vi "3_2_Face_Detection_Inference(CPU,GPU,RT)(File).vi"() -> ()   [LabVIEW 2020]
doc: "This example demonstrates the usage of the \"DeepLTK FPGA Addon\" for deploying a Face Detection model on a PXI-FPGA board, utilizing an input image sourced from a file.\n\nMore Examples: https://github.com/ngenehub/deepltk_fpga_examples"
uses:
  <vilib>/Ngene/Deep Learning Toolkit/Toolkit/NN_Network/Controls/NN_Device.ctl
  <vilib>/Ngene/Deep Learning Toolkit/Toolkit/NN_Network/Controls/NN_Save_Before_Destroy_Options.ctl
  6caafd12-b030-411a-8c32-73dfdbcc6777.vi
  <vilib>/Ngene/Deep Learning Toolkit/Toolkit/Utils/Vision/Coords_Rect2PolyLine.vi
  <vilib>/Ngene/Deep Learning Toolkit/Toolkit/NN_Network/API/NN_Set_Input/3D/NN_Set_Input(3D_SGL_idx).vi
  <vilib>/vision/NI_Vision_Development_Module.lvlib
  <vilib>/Ngene/Deep Learning Toolkit/Toolkit/Deep_Learning_Toolkit_by_Ngene.lvlib
  <vilib>/ptbypt/NI_PtbyPt.lvlib
panel:
  out "Loop time":dbl=0.10532894999996642 format="%#_4p"
  in  "NN_Device":T1
  out "Display":T2(plugin-control)
  out "Inference time":dbl=0.09766583999989961 format="%#_4p"
  out "Sample Path":path=path "D:/Ngene/GitHub/deepltk_fpga_examples/2_Face_Detection(PXI,sbRIO)/Dataset/Images/8_Election_Campain_Election_Campaign_8_529.jpg"
  in  "Select Sample":i32=19 min=0 max=19 step=1
  in  "Dataset Path (Images)":path=path "D:/Ngene/GitHub/deepltk_fpga_examples/2_Face_Detection(PXI,sbRIO)/Dataset/Images"
  in  "Confidence_Thresh":sgl=0.4
  in  "IOU_Thresh":sgl=0.3
  in  "Stop":bool
  in  "Weight File Path":path=path "D:/Ngene/GitHub/deepltk_fpga_examples/2_Face_Detection(PXI,sbRIO)/Models/Face_Detection_Original/Face_Detection.bin"
  in  "Configuration File Path":path=path "D:/Ngene/GitHub/deepltk_fpga_examples/2_Face_Detection(PXI,sbRIO)/Models/Face_Detection_Original/Face_Detection.cfg"
  # "Overview: \nOverview:  This example demonstrates usage of Deep Learning Toolkit for deploying a Face Detection model, utilizing an input image sourced from a file.\nRequirements: \n•DeepLTK - Deep Learning Toolkit for LabVIEW (https://www.ngene.co/deep-learning-toolkit-for-labview)\n• NI Vision Development Module"
  # "Instructions:\nNote: To run the example on an RT target, copy the pretrained model and test images to the RT target.\n1. Provide the \"Network Configuration File Path\" and \"Weight File Path\" locted in \"Models\\Face_Detection_Original\" folder in the project.\n2.\tProvide the path to the folder with test images in the \"Dataset Path (Images)\" control. A sample is available in the \"Dataset\" folder. \n3. Use NN_Device to specify the device (CPU or GPU) for execution. GPU is applicable only for 64-bit LabVIEW.\n4. Run the VI. \n5. Observe the detections drawn on the \"Display\". The info on the top left of each bounding box represents detected object class and the confidence level.  \n4. Change \"Select Sample\" value to select different image samples from the datset.\n5. Hit \"Stop\" button to stop the VI\nMore Examples:  https://github.com/ngenehub/deepltk_examples"
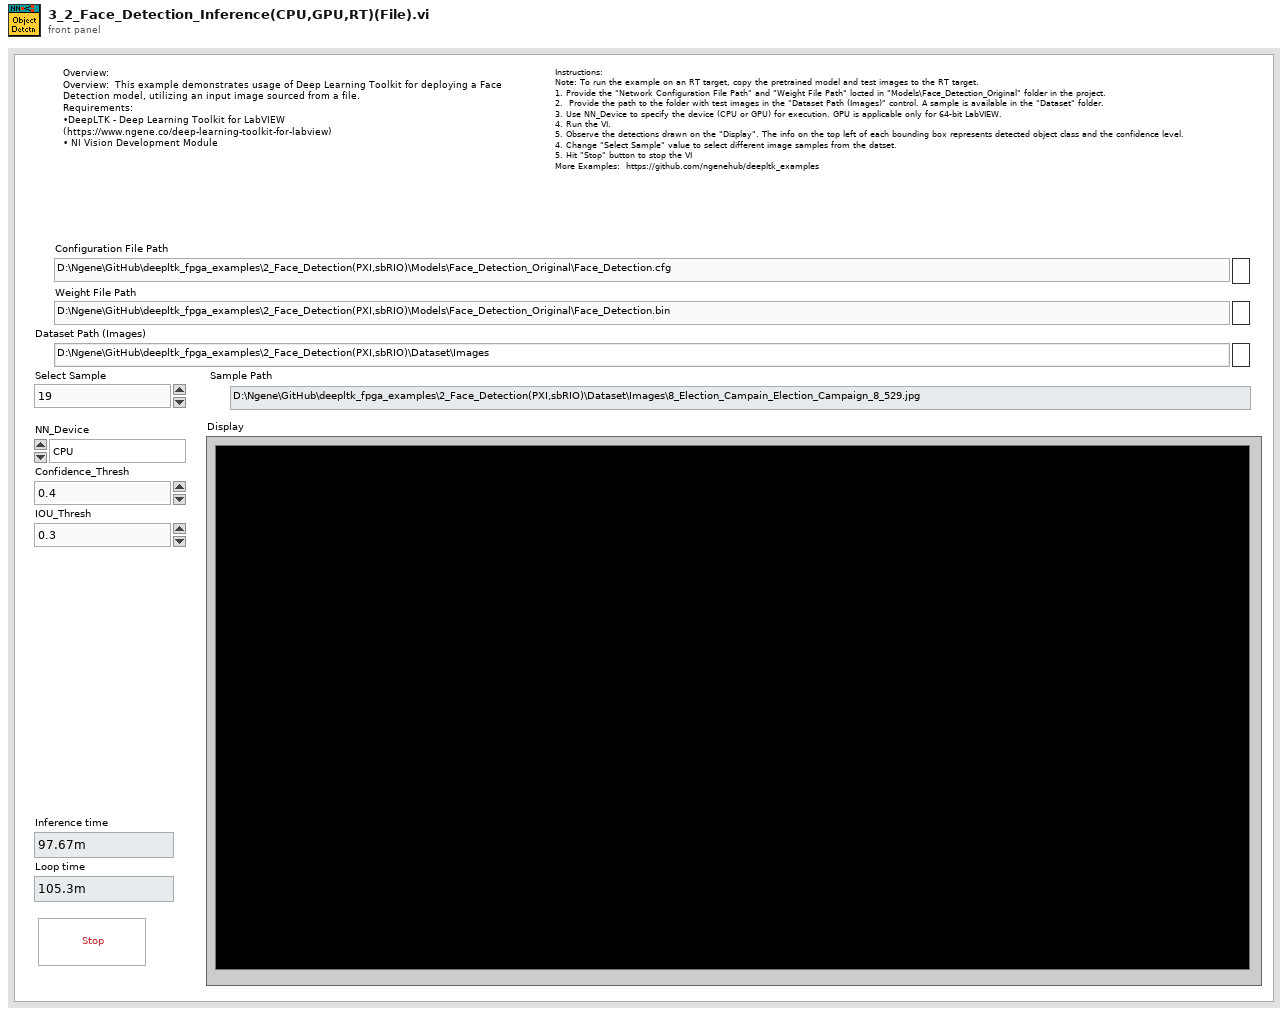
[diagram p1: front panel]
types:
  T1 = typedef "Deep_Learning_Toolkit_by_Ngene.lvlib/NN_Device.ctl" = enum16{"CPU", "GPU"}
  T2 = typedef "IMAQ Image.ctl" = refnum<image>
  T3 = typedef "Image Type" = u32
  T4 = typedef "Deep_Learning_Toolkit_by_Ngene.lvlib/NN_Save_Before_Destroy_Options.ctl" = cluster{"CFG?":bool, "Weights?":bool, "Render?":bool}
  T5 = typedef "Deep_Learning_Toolkit_by_Ngene.lvlib/NN_Config_Params.ctl" = cluster{"Name":string, "mBatch":i32, "NN_Train_Params":T6, "LR_Decay_Policy":T9, "Labels":string[], "Loss":T11}
  T6 = typedef "Deep_Learning_Toolkit_by_Ngene.lvlib/NN_Train_Params.ctl" = cluster{"Optimizer":T7, "Beta_1":sgl, "Beta_2":sgl, "Weight Decay(L1)":sgl, "Weight Decay(L2)":sgl, "Data_Sampling":T8}
  T7 = typedef "Deep_Learning_Toolkit_by_Ngene.lvlib/NN_Train_Optimizer.ctl" = enum16{"SGD", "Adam", "Adagrad", "Adadelta", "RMSProp", "Nesterov"}
  T8 = typedef "Deep_Learning_Toolkit_by_Ngene.lvlib/NN_Train_Data_Sampling.ctl" = enum16{"Random", "Sequential"}
  T9 = typedef "Deep_Learning_Toolkit_by_Ngene.lvlib/NN_LR_Policy_Cfg.ctl" = cluster{"Policy_Type":T10, "LR0":dbl, "k":sgl, "WarmUp_Policy":enum16{"Step", "Ramp"}, "WarmUp_Iter":i32, "WarmUp_Ratio":sgl}
  T10 = typedef "Deep_Learning_Toolkit_by_Ngene.lvlib/NN_LR_Policy_Type.ctl" = enum16{"Manual", "Step", "Exp", "1/t"}
  T11 = typedef "Deep_Learning_Toolkit_by_Ngene.lvlib/NN_Loss_Config_Params.ctl" = cluster{"Loss_Type":T12, "Loss_Conf_Params":variant}
  T12 = typedef "Deep_Learning_Toolkit_by_Ngene.lvlib/NN_Loss_Type.ctl" = enum16{"None", "MSE", "CrossEntropy", "YOLO_v2", "YOLO_v4"}
  T13 = typedef "Deep_Learning_Toolkit_by_Ngene.lvlib/NN_Layer_Config_Params.ctl" = cluster{"Layer_Type":T14, "Layer_Conf_Params":variant, "Input Layers":string[]}
  T14 = typedef "Deep_Learning_Toolkit_by_Ngene.lvlib/NN_Layer_Type.ctl" = enum16{"Input1D", "Input3D", "Conv1D", "Conv2D", "Conv2D_Adv", "MaxPool", "AvgPool", "UpSample", "DropOut3D", "ShortCut", "Concat", "SoftMax3D", "FC", "DropOut", "Softmax", "Flatten", "YOLO_v2", "YOLO_v4", "Activation", "BatchNormalization", "Unsupported"}
  T15 = typedef "Deep_Learning_Toolkit_by_Ngene.lvlib/NN.ctl" = cluster{"Name":string, "No of Layers":i32, "mBatch":i32, "Layers":T16[], "Dimty":T17, "Dims_In":T18, "Dims_Out":T18, "Working_Dir":path, "Train?":bool, "Train_Params":T6, "LR_Update_Policy":T9, "Session Data":T19, "Ground_truth":T20, "NNg_hdls":T21, "NN_Device":T1, "GPU Id":i32, "Labels":string[], "Receptive Field":T22[], "Loss_Type":T12, "Loss_Cfg_Prms":variant, "NNG_WS":T23}
  T16 = typedef "Deep_Learning_Toolkit_by_Ngene.lvlib/NN_Layer_ref.ctl" = refnum<data-value>
  T17 = typedef "Deep_Learning_Toolkit_by_Ngene.lvlib/NN_In_Out_Dim-ty.ctl" = enum8{"In1D_Out1D", "In3D_Out1D", "In3D_Out3D", "In3D_OutBBox"}
  T18 = typedef "Deep_Learning_Toolkit_by_Ngene.lvlib/NN_Dims(C,H,W).ctl" = cluster{"C":i32, "H":i32, "W":i32}
  T19 = typedef "Deep_Learning_Toolkit_by_Ngene.lvlib/NN_Train_Session_Data.ctl" = cluster{"Epochs":sgl, "Tot_Iter":i32, "LR":sgl, "LR_iter":i32}
  T20 = typedef "Deep_Learning_Toolkit_by_Ngene.lvlib/NN_Ground_truth.ctl" = cluster{"Y":variant}
  T21 = typedef "Deep_Learning_Toolkit_by_Ngene.lvlib/nng_cuda_handles.ctl" = cluster{"cudnn":u64, "cublas":u64, "stream":u64, "curand":u64}
  T22 = typedef "Deep_Learning_Toolkit_by_Ngene.lvlib/NN_Dims(V,H).ctl" = cluster{"V":i32, "H":i32}
  T23 = typedef "Deep_Learning_Toolkit_by_Ngene.lvlib/NNG_WS.ctl" = cluster{"NNG_WS_Mem":T24, "Max_WS_Size":i64}
  T24 = typedef "Deep_Learning_Toolkit_by_Ngene.lvlib/NNg_WS_Mem_DVR.ctl" = refnum<data-value>
  T25 = typedef "Deep_Learning_Toolkit_by_Ngene.lvlib/NN_Layer.ctl" = cluster{"Name":string, "Layer_Data":variant, "Layer_Type":T14, "Dims_In":T18, "Layers_In":variant, "Dims_Out":T18, "Layers_Out":variant, "Metrics":T26, "GPU_Data":variant, "mBatch":i32, "NN_Device":T1, "NNg_hdls":T21, "Train?":bool, "Dimty":T27, "RecptField":T28}
  T26 = typedef "Deep_Learning_Toolkit_by_Ngene.lvlib/NN_Layer_Metrics.ctl" = cluster{"Data":dbl, "Params":dbl, "Ops":dbl}
  T27 = typedef "Deep_Learning_Toolkit_by_Ngene.lvlib/NN_Layer_Dimty.ctl" = enum16{"1D", "3D"}
  T28 = typedef "Deep_Learning_Toolkit_by_Ngene.lvlib/NN_Layer_RF_State.ctl" = cluster{"Dims":T22, "J":T22}
  T29 = typedef "Deep_Learning_Toolkit_by_Ngene.lvlib/NN_BBox_Detection.ctl" = cluster{"Class":i32, "Conf Level":sgl, "BBox":T30}
  T30 = typedef "Deep_Learning_Toolkit_by_Ngene.lvlib/NN_BBox.ctl" = cluster{"x":sgl, "y":sgl, "w":sgl, "h":sgl}
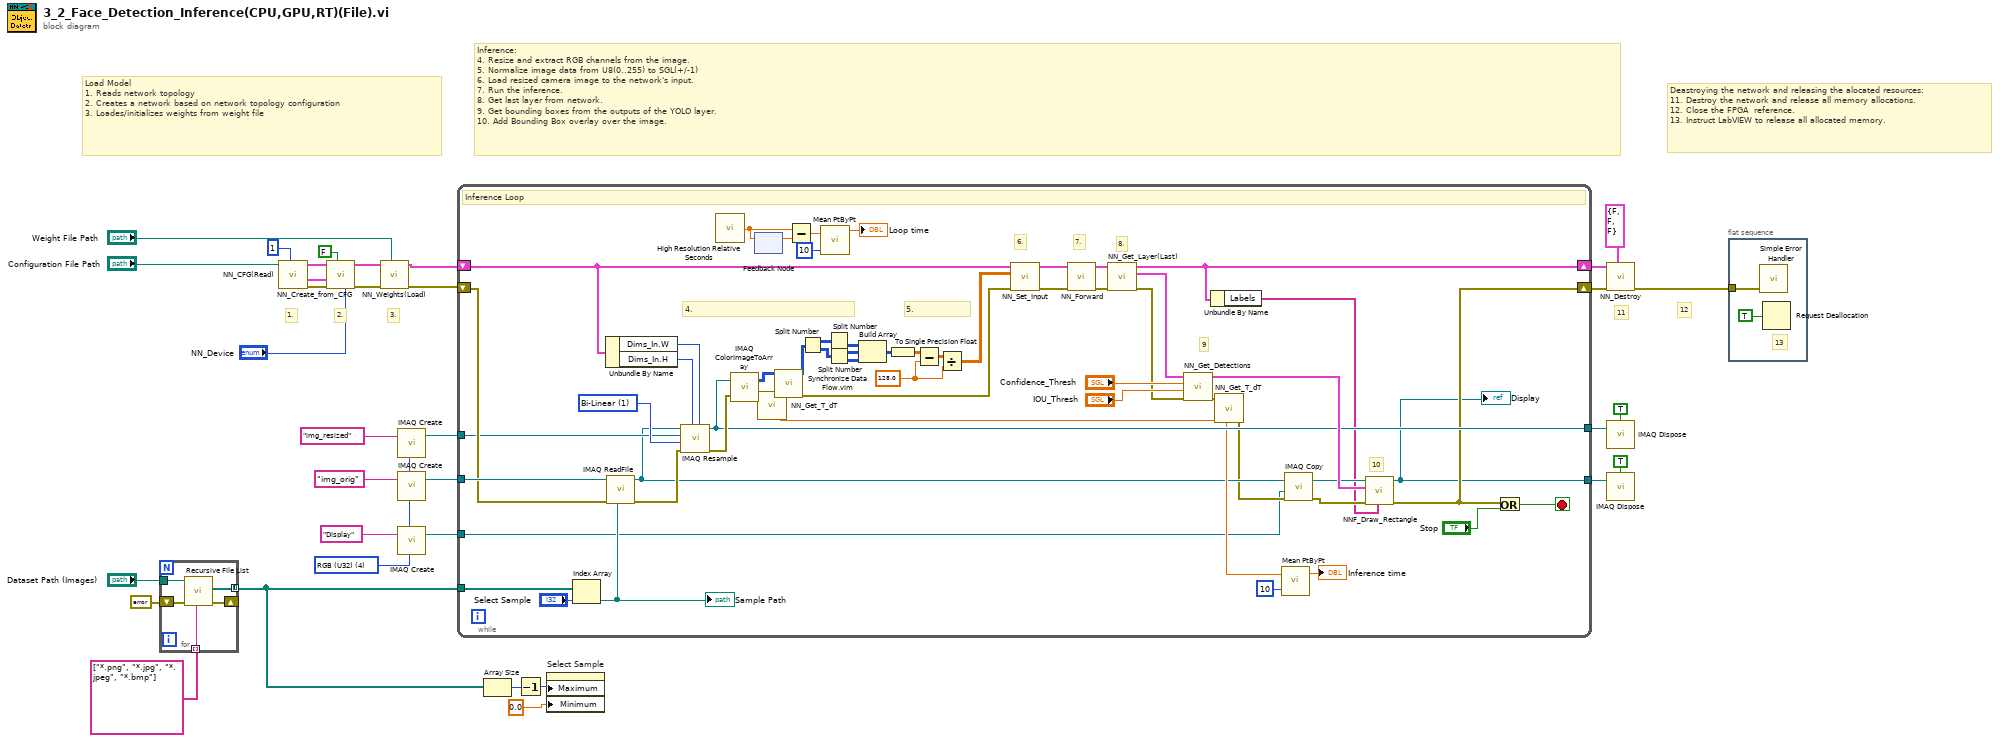
[diagram p0: block diagram]
diagram:
  w2 = T3 4 items=["Grayscale (U8)", "Grayscale (I16)", "Grayscale (SGL)", "Complex (CSG)", "RGB (U32)", "HSL (U32)", "RGB (U64)", "Grayscale (U16)"] ("Image Type")
  # "3."
  # "2."
  # "1."
  # "12"
  # "11"
  # "Deastroying the network and releasing the alocated resources: \n11. Destroy the network and release all memory allocations.\n12. Close the FPGA  reference.\n13. Instruct LabVIEW to release all allocated memory."
  # "Inference:\n4.\tResize and extract RGB channels from the image.\n5.\tNormalize image data from U8(0..255) to SGL(+/-1)\n6.\tLoad resized camera image to the network's input.\n7.\tRun the inference.\n8.\tGet last layer from network.\n9.\tGet bounding boxes from the outputs of the YOLO layer. \n10.\tAdd Bounding Box overlay over the image."
  # "Load Model\n1.\tReads network topology\n2.\tCreates a network based on network topology configuration\n3.\tLoades/initializes weights from weight file"
  n1 = for {
    tunnel: "Dataset Path (Images)" -> [w39]
    tunnel: string[] ["*.png", "*.jpg", "*.jpeg", "*.bmp"] ("pattern") -> [w38] mode=indexing
    tunnel: [w37] -> w26 mode=concatenating
    shift-right: [w35] -> _
    shift-left: errorcluster {"status"=FALSE, "code"=0, "source"=""} ("error out") -> [w36]
    n2 = call <vilib>:"Recursive File List.vi"("pattern"=w38, "error in (no error)"=w36, "Folder Path"=w39) -> ("error out"=w35:errorcluster, "All Files in Dir"=w37:path[])  [unwired: 4 in, 3 out]
  }
  n3 = call <vilib>:"NN_CFG(Read).vi"("mBatch"=1, "CFG file path"="Configuration File Path") -> ("error out"=w15:errorcluster, "Net_Cfg"=w11:T5, "Layer_Cfg"=w16:T13[])  [unwired: 7 in]
  n4 = call <vilib>:"NN_Create_from_CFG.vi"("NN_Device"="NN_Device", "Train? (false)"=FALSE ("Train?"), "error in (no error)"=w15, "Net_Cfg"=w11, "Layer_Cfg"=w16) -> ("error out"=w14:errorcluster, "NN out"=w13:T15)  [unwired: 5 in]
  n5 = call <vilib>:"NN_Weights(Load).vi"("Weight File Path"="Weight File Path", "error in (no error)"=w14, "NN in"=w13) -> ("error out"=w8:errorcluster, "NN out"=w9:T15)  [unwired: 7 in]
  n6 = call "IMAQ Create"("Image Name"="img_resized", "Image Type"=w2) -> ("New Image"=w22:T2)  [unwired: 3 in, 1 out]
  n7 = call "IMAQ Create"("Image Name"="img_orig", "Image Type"=w2) -> ("New Image"=w30:T2)  [unwired: 3 in, 1 out]
  n8 = call "IMAQ Create"("Image Name"="Display", "Image Type"=w2) -> ("New Image"=w1:T2)  [unwired: 3 in, 1 out]
  n9 = while {
    shift-right: [w42] -> w19
    shift-left: w9 -> [w79]
    tunnel: [w47] -> w34
    tunnel: w26 -> [w93]
    tunnel: w30 -> [w90]
    shift-right: [w48] -> w29
    shift-left: w8 -> [w87]
    tunnel: w22 -> [w78]
    tunnel: [w77] -> w20
    tunnel: w1 -> [w40]
    stop <- w96 stop-if-true
    w66 = sgl 128.0
    w92 = u32 1 items=["Zero Order", "Bi-Linear", "Quadratic", "Cubic Spline"] ("Interpolation Type")
    # "5."
    # "4."
    # "7."
    # "6."
    # "10"
    # "9"
    # "8."
    # "Inference Loop"
    n10 = Index Array(array=w93, index="Select Sample") -> (element=w82:path)
    "Sample Path" <- w82
    n11 = Unbundle By Name(w79) -> ("Dims_In.W"=w89:i32, "Dims_In.H"=w88:i32)
    n12 = call "IMAQ ReadFile"("File Path"=w82, "error in (no error)"=w87, "Image"=w90) -> ("error out"=w81:errorcluster, "Image Out"=w45:T2)  [unwired: 4 in, 3 out]
    n13 = call "IMAQ Resample"("X Resolution"=w89, "Y Resolution"=w88, "error in (no error)"=w81, "Interpolation Type"=w92, "Image Dst"=w78, "Image Src"=w45) -> ("error out"=w80:errorcluster, "Image Dst Out"=w77:T2)  [unwired: 4 in]
    n14 = call <vilib>:"High Resolution Relative Seconds.vi"() -> ("relative seconds"=w53:dbl)
    n15 = call "IMAQ ColorImageToArray"("Image"=w77, "error in (no error)"=w80) -> ("Image Pixels (U32)"=w59:u32[][], "error out"=w61:errorcluster)  [unwired: 2 in, 1 out]
    n16 = feedback-in #1(w53) -> ()
    n17 = feedback #1() -> (w52:dbl)  [unwired: 1 in]
    n18 = call <vilib>:"NN_Get_T_dT.vi"("error in (no error)"=w61) -> ("T_out"=w56:dbl, "error out"=w57:errorcluster)  [unwired: 6 in, 1 out]
    n19 = call "Synchronize Data Flow.vim"("input 4"=w57, "input 1"=w59) -> ("output 4"=w60:errorcluster, "output 1"=w58:u32[][])  [unwired: 2 in, 2 out]
    n20 = Subtract(x=w53, y=w52) -> (x-y=w51:dbl)
    n21 = Split Number(x=w58) -> (hi(x)=w70:u16[][], lo(x)=w69:u16[][])
    n22 = call <vilib>:"Mean PtByPt.vi"("x"=w51, "sample length"=10) -> ("mean"=→"Loop time":dbl)  [unwired: 2 in, 1 out]
    n23 = Split Number(x=w70) -> (lo(x)=w71:u8[][])  [unwired: 1 out]
    n24 = Split Number(x=w69) -> (hi(x)=w72:u8[][], lo(x)=w73:u8[][])
    n25 = Build Array(w71, w72, w73) -> (w74:u8[][][])
    n26 = To Single Precision Float(number=w74) -> (single precision float=w67:sgl[][][])
    n27 = Subtract(x=w67, y=w66) -> (x-y=w68:sgl[][][])
    n28 = Divide(x=w68, y=w66) -> (x/y=w65:sgl[][][])
    n29 = call-poly <vilib>:"NN_Set_Input.vi"("error in (no error)"=w60, "Data_In(3D_SGL)"=w65, "NN in"=w79) -> ("error out"=w85:errorcluster, "NN out"=w86:T15)  [unwired: 7 in]
    n30 = call <vilib>:"NN_Forward.vi"("error in (no error)"=w85, "NN in"=w86) -> ("error out"=w76:errorcluster, "NN out"=w63:T15)  [unwired: 6 in, 2 out]
    n31 = call <vilib>:"NN_Get_Layer(Last).vi"("error in (no error)"=w76, "NN in"=w63) -> ("error out"=w64:errorcluster, "Last_Layer"=w62:T25, "NN out"=w42:T15)  [unwired: 6 in, 1 out]
    n32 = call <vilib>:"NN_Get_Detections.vi"("error in"=w64, "IOU_Thrsh"="IOU_Thresh", "Confidence_Thrsh"="Confidence_Thresh", "YOLO_Layer"=w62) -> ("error out"=w83:errorcluster, "Detections"=w84:T29[])  [unwired: 6 in]
    n33 = Unbundle By Name(w42) -> ("Labels"=w41:string[])
    n34 = call <vilib>:"NN_Get_T_dT.vi"("T_in"=w56, "error in (no error)"=w83) -> ("error out"=w44:errorcluster, "dT"=w55:dbl)  [unwired: 5 in, 1 out]
    n35 = call <vilib>:"Mean PtByPt.vi"("x"=w55, "sample length"=10) -> ("mean"=→"Inference time":dbl)  [unwired: 2 in, 1 out]
    n36 = call "IMAQ Copy"("error in (no error)"=w44, "Image Dst"=w40, "Image Src"=w45) -> ("error out"=w43:errorcluster, "Image Dst Out"=w46:T2)  [unwired: 3 in]
    n37 = call "NNF_Draw_Rectangle.vi"("Labels"=w41, "error in (no error)"=w43, "Draw_Boxes"=w84, "Img in"=w46) -> ("error out"=w48:errorcluster, "Img out"=w47:T2)  [unwired: 6 in]
    "Display" <- w47
    n38 = Or(x=w48, y="Stop") -> (x .or. y?=w96:bool)
  }
  n39 = Array Size(array=w26) -> (size(s)=w27:i32)
  n40 = Decrement(x=w27) -> (x-1=w25:i32)
  n41 = property on="Select Sample" class="DigNum (strict)"("Maximum"=w25, "Minimum"=0.0 ("Data Entry Limits:Minimum")) -> ()  [unwired: 2 in, 2 out]
  n42 = call <vilib>:"NN_Destroy.vi"("Save (T, T, T)"=T4 {"CFG?"=FALSE, "Weights?"=FALSE, "Render?"=FALSE}, "error in (no error)"=w29, "NN in"=w19) -> ("error out"=w18:errorcluster)  [unwired: 7 in, 1 out]
  n43 = call "IMAQ Dispose"("All Images? (No)"=TRUE, "Image"=w20) -> ()  [unwired: 4 in, 1 out]
  n44 = call "IMAQ Dispose"("All Images? (No)"=TRUE, "Image"=w34) -> ()  [unwired: 4 in, 1 out]
  n45 = flat-sequence {
    tunnel: w18 -> [w98]
    frame #0 {
      # "13"
      n46 = call <vilib>:"Simple Error Handler.vi"("error in (no error)"=w98) -> ()  [unwired: 4 in, 5 out]
      n47 = Request Deallocation(TRUE ("flag")) -> ()
    }
  }
